vi "Generate Initialize Finish Event.vi"(8 "error in (no error)":errorcluster) -> (0 "error out":errorcluster)   [LabVIEW 2019, in "FootScan Engine.lvlib"]
uses:
  FootScan Engine.lvlib
panel:
  # "Input"
  # "Output"
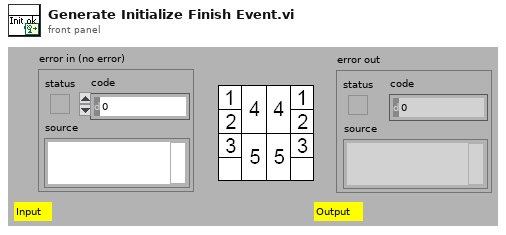
[diagram p1: front panel]
types:
  T1 = typedef "Event Message.lvlib/Event.ctl" = refnum<user-event>
  T2 = cluster{"Name":string, string, "variant":variant}
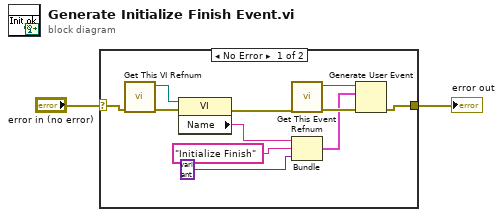
[diagram p0: block diagram]
diagram:
  n1 = case shown="No Error" "error in (no error)" {
    selector: "error in (no error)" -> [w13 w14]
    tunnel: [w7 w14] -> w1
    frame No Error {
      n2 = call "Get This VI Refnum.vi"("error in (no error)"=w13) -> ("error out"=w11:errorcluster, "This VI Refnum Out"=w12:refnum<vi>)  [unwired: 9 in]
      n3 = property class="VI"(reference=w12, error in=w11) -> (error out=w9:errorcluster, "Name"=w6:string)  [unwired: 1 out]
      n4 = call "Get This Event Refnum.vi"("error in (no error)"=w9) -> ("error out"=w8:errorcluster, "This Event Refnum Out"=w10:T1)  [unwired: 9 in]
      n5 = Bundle("Name"=w6, "Initialize Finish", "variant"=variant) -> (w3:T2)  [unwired: 1 in]
      n6 = Generate User Event(user event=w10, event data cluster=w3, error in=w8) -> (error out=w7:errorcluster)  [unwired: 1 in, 1 out]
    }
    frame Error {
    }
  }
  "error out" <- w1
